vi "enumerateStaticDependencies.vi"(8 "error in (no error)":errorcluster, 11 "GUI":refnum<class "GUI.lvclass">) -> (0 "error out":errorcluster, 2 "Static Dependencies":refnum<class "Dependency.lvclass">[](array[class]), 3 "GUI out":refnum<class "GUI.lvclass">)   [LabVIEW 2022 SP3, in "GUI.lvclass"]
uses:
  GUI.lvclass
  <vilib>/JKI/JKI SMO/Dependency/Dependency.lvclass
  DB2/DB2.lvclass
  Analyzer/Analyzer.lvclass
  Home/Home.lvclass
  <vilib>/Utility/Data Type/Get Cluster Information.vi
  <vilib>/Utility/Data Type/Get Type Information.vi
  <vilib>/JKI/JKI SMO/SMO.UI/SMO.UI.lvclass
  <vilib>/JKI/JKI SMO/SMO/SMO.lvclass
panel:
  # "For instructions on how to use the JKI State Machine Objects, examples and video tutorials, visit:\nhttp://jki.net/state-machine-objects/\n\nJKI State Machine Objects™\nhttp://jki.net/state-machine-objects/\nCopyright (C) 2005-2015, JKI <info@jki.net>\nALL RIGHTS RESERVED"
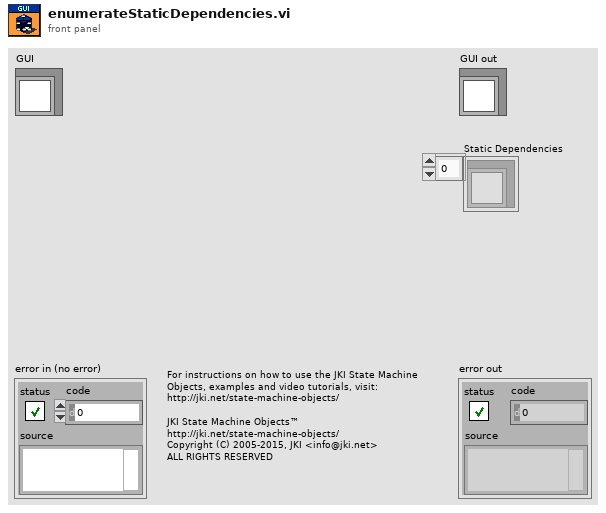
[diagram p1: front panel]
types:
  T1 = cluster{"DB2":refnum<class "DB2.lvclass">, "Analyzer":refnum<class "Analyzer.lvclass">, "Home":refnum<class "Home.lvclass">}
  T2 = cluster{"First":refnum<class "SMO.lvclass">, "Second":refnum<class "SMO.lvclass">}
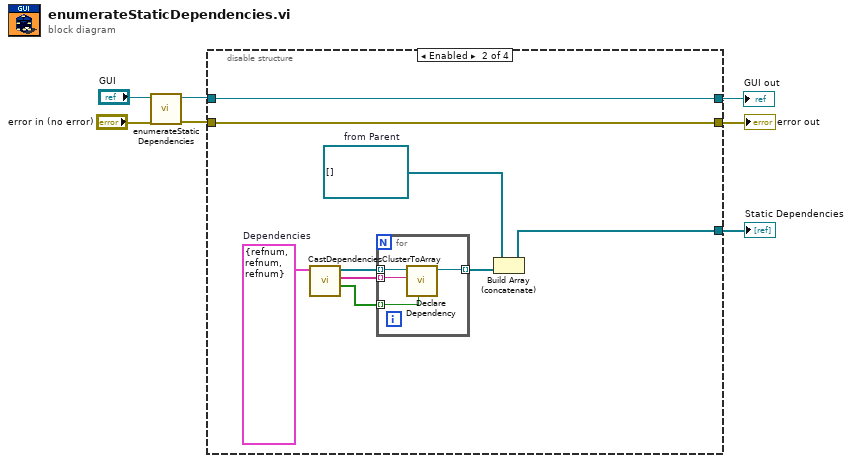
[diagram p0: block diagram]
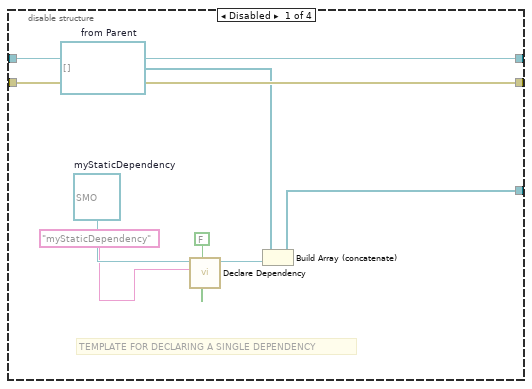
[diagram p2: hidden frame]
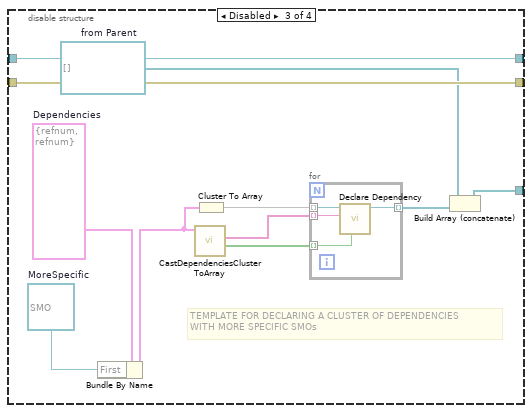
[diagram p3: hidden frame]
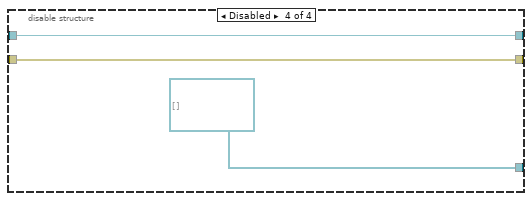
[diagram p4: hidden frame]
diagram:
  n1 = call-parent "enumerateStaticDependencies.vi"("error in (no error)"="error in (no error)", "SMO"="GUI") -> ("error out"=w6:errorcluster, "SMO out"=w7:refnum<class "GUI.lvclass">)  [unwired: 7 in, 1 out]
  n2 = disable-structure shown="Enabled" {
    disable-tunnel: w7 -> [w15 w24 w39 w46]
    disable-tunnel: [w15 w24 w39 w46] -> w4
    disable-tunnel: w6 -> [w14 w23 w38 w45]
    disable-tunnel: [w14 w23 w38 w45] -> w1
    disable-tunnel: [w9 w21 w36 refnum<class "Dependency.lvclass">[] [] ("appended array")] -> w2
    frame Disabled {
      w8 = refnum<class "Dependency.lvclass">[] []  # from Parent
      w13 = refnum<class "SMO.lvclass"> refnum  # myStaticDependency
      # "TEMPLATE FOR DECLARING A SINGLE DEPENDENCY"
      n3 = call <vilib>:"Declare Dependency.vi"("Shared Resource (F)"=FALSE, "Name"="myStaticDependency", "Type"=w13) -> ("Dependency out"=w10:refnum<class "Dependency.lvclass">)  [unwired: 7 in, 1 out]
      n4 = Build Array (concatenate)(w8, w10) -> (w9:refnum<class "Dependency.lvclass">[])
    }
    frame Enabled {
      w19 = T1 {"DB2"=refnum, "Analyzer"=refnum, "Home"=refnum}  # Dependencies
      w20 = refnum<class "Dependency.lvclass">[] []  # from Parent
      n5 = call <vilib>:"CastDependenciesClusterToArray.vi"("Dependencies Cluster"=w19) -> ("Shared Resources"=w16:bool[], "Dependencies Names"=w17:string[], "Dependencies Array"=w18:refnum<class "SMO.lvclass">[])  [unwired: 8 in]
      n6 = for {
        tunnel: [w28] -> w22 mode=indexing
        tunnel: w18 -> [w27] mode=indexing
        tunnel: w17 -> [w26] mode=indexing
        tunnel: w16 -> [w25] mode=indexing
        n7 = call <vilib>:"Declare Dependency.vi"("Shared Resource (F)"=w25, "Name"=w26, "Type"=w27) -> ("Dependency out"=w28:refnum<class "Dependency.lvclass">)  [unwired: 7 in, 1 out]
      }
      n8 = Build Array (concatenate)(w20, w22) -> (w21:refnum<class "Dependency.lvclass">[])
    }
    frame Disabled {
      w31 = refnum<class "SMO.lvclass"> refnum  # MoreSpecific
      w32 = T2 {"First"=refnum, "Second"=refnum}  # Dependencies
      w35 = refnum<class "Dependency.lvclass">[] []  # from Parent
      # "TEMPLATE FOR DECLARING A CLUSTER OF DEPENDENCIES\nWITH MORE SPECIFIC SMOs"
      n9 = Bundle By Name(cluster=w32, "First"=w31) -> (w29:T2)
      n10 = call <vilib>:"CastDependenciesClusterToArray.vi"("Dependencies Cluster"=w29) -> ("Shared Resources"=w33:bool[], "Dependencies Names"=w34:string[])  [unwired: 8 in, 1 out]
      n11 = Cluster To Array(cluster=w29) -> (array=w30:refnum<class "SMO.lvclass">[])
      n12 = for {
        tunnel: [w43] -> w37 mode=indexing
        tunnel: w30 -> [w42] mode=indexing
        tunnel: w34 -> [w41] mode=indexing
        tunnel: w33 -> [w40] mode=indexing
        n13 = call <vilib>:"Declare Dependency.vi"("Shared Resource (F)"=w40, "Name"=w41, "Type"=w42) -> ("Dependency out"=w43:refnum<class "Dependency.lvclass">)  [unwired: 7 in, 1 out]
      }
      n14 = Build Array (concatenate)(w35, w37) -> (w36:refnum<class "Dependency.lvclass">[])
    }
    frame Disabled {
    }
  }
  "error out" <- w1
  "GUI out" <- w4
  "Static Dependencies" <- w2
